vi "notemaker.vi"(11 "project-param in":T1) -> (3 "Reaper Note":string)   [LabVIEW 2019]
uses:
  Project Parameters.ctl
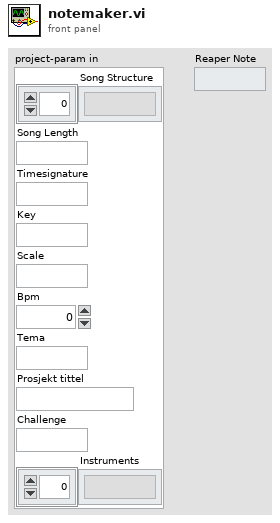
[diagram p1: front panel]
types:
  T1 = typedef "Project Parameters.ctl" = cluster{"Song Structure":string[], "Song Length":string, "Timesignature":string, "Key":string, "Scale":string, "Bpm":i32, "Tema":string, "Prosjekt tittel":string, "Challenge":string, "Instruments":string[]}
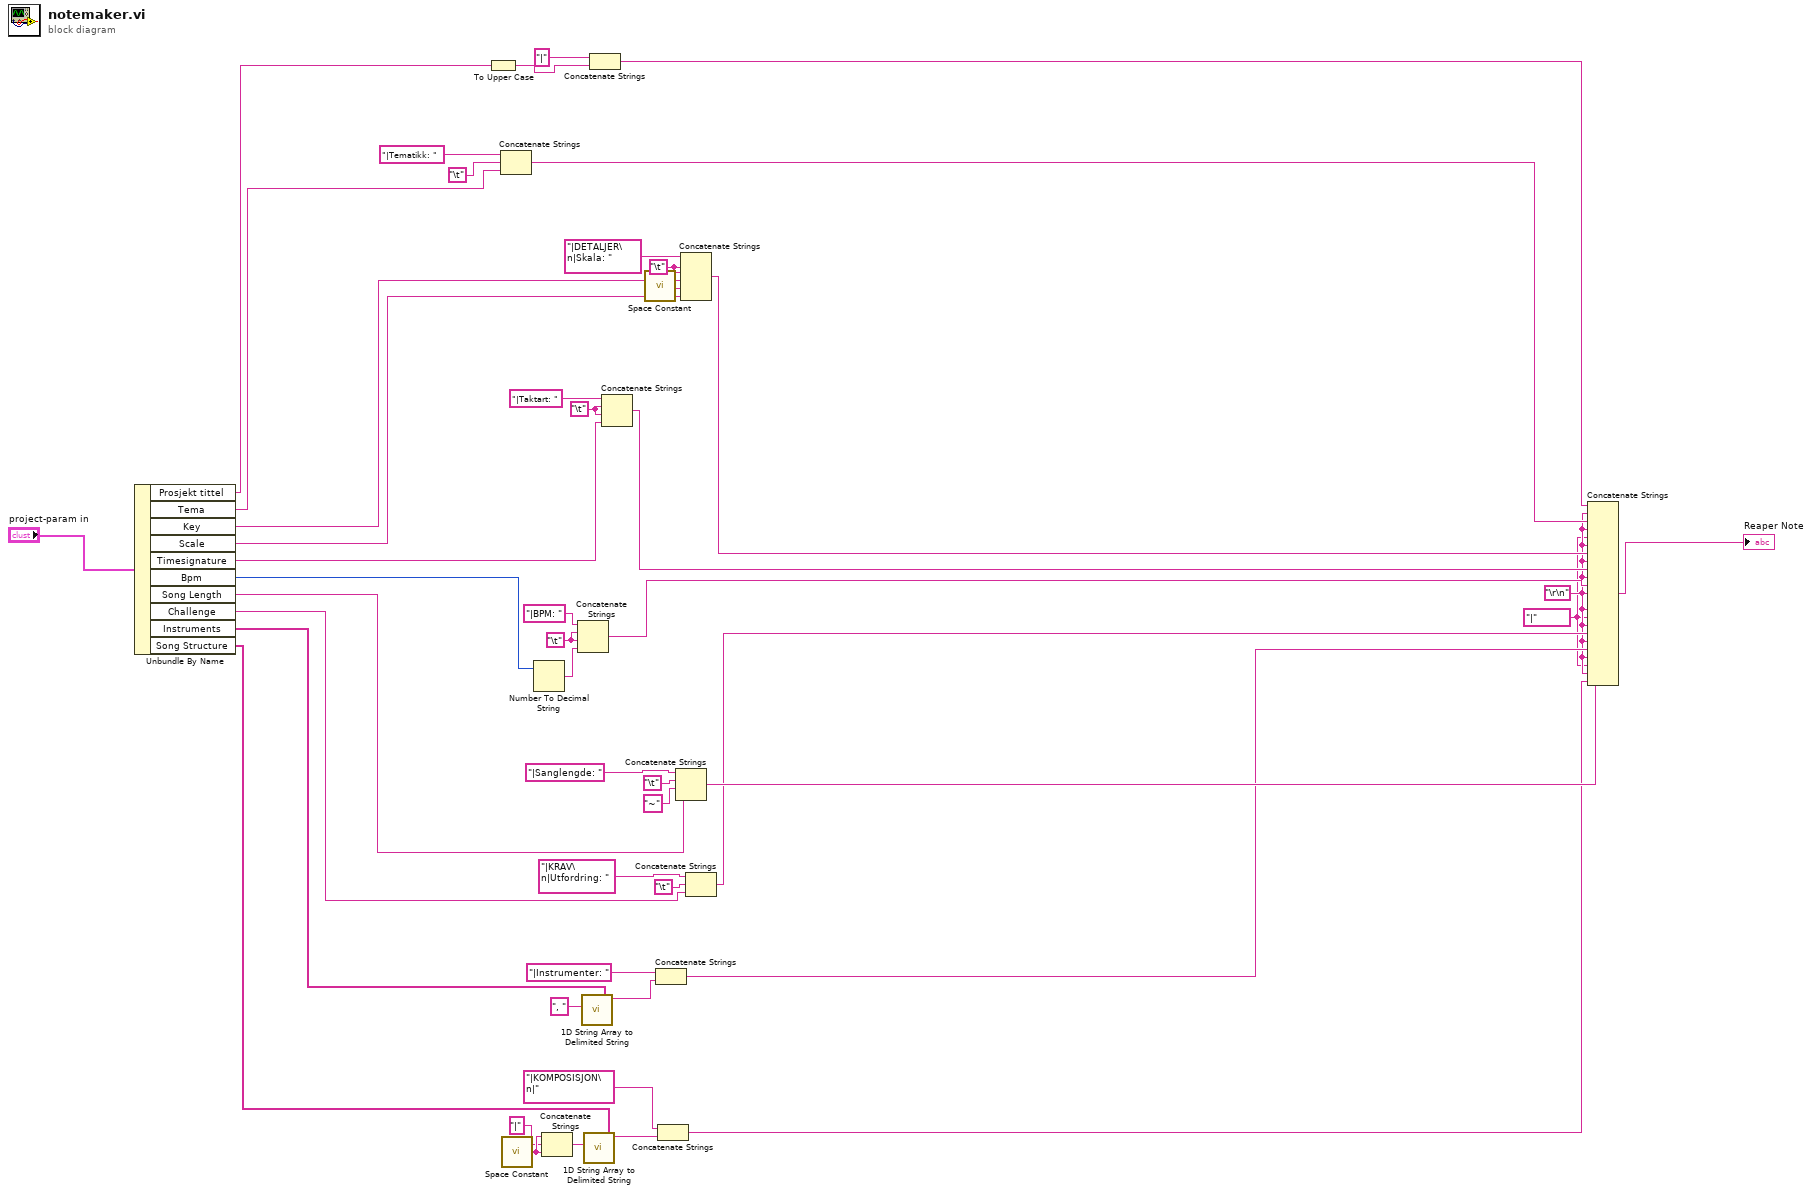
[diagram p0: block diagram]
diagram:
  w4 = "\t"
  w2 = "\t"
  w3 = "\t"
  w9 = "|" ("string")
  w10 = "\r\n"
  n1 = Unbundle By Name("project-param in") -> ("Prosjekt tittel"=w36:string, "Tema"=w11:string, "Key"=w33:string, "Scale"=w32:string, "Timesignature"=w31:string, "Bpm"=w46:i32, "Song Length"=w29:string, "Challenge"=w26:string, "Instruments"=w21:string[], "Song Structure"=w14:string[])
  n2 = To Upper Case(1:w36) -> (0:w37:string)
  n3 = Concatenate Strings("|Tematikk: " ("string"), "\t", w11) -> (w34:string)
  n4 = call <vilib>:"Space Constant.vi"() -> ("String"=w19:string)
  n5 = Number To Decimal String(number=w46) -> (decimal integer string=w47:string)  [unwired: 1 in]
  n6 = Concatenate Strings(w19, "|" ("string"), w19) -> (w20:string)
  n7 = Concatenate Strings("|BPM: " ("string"), w4, w4, w47) -> (w48:string)
  n8 = call <vilib>:"1D String Array to Delimited String.vi"("delimiter"=", " ("string"), "string array"=w21) -> ("delimited string"=w22:string)  [unwired: 9 in]
  n9 = call <vilib>:"1D String Array to Delimited String.vi"("delimiter"=w20, "string array"=w14) -> ("delimited string"=w15:string)  [unwired: 9 in]
  n10 = Concatenate Strings("|" ("string"), w37) -> (w13:string)
  n11 = Concatenate Strings("|Taktart: ", w3, w3, w31) -> (w43:string)
  n12 = call <vilib>:"Space Constant.vi"() -> ("String"=w40:string)
  n13 = Concatenate Strings("|Instrumenter: " ("string"), w22) -> (w23:string)
  n14 = Concatenate Strings("|KOMPOSISJON\n|" ("string"), w15) -> (w8:string)
  n15 = Concatenate Strings("|Sanglengde: " ("string"), "\t", "~" ("string"), w29) -> (w28:string)
  n16 = Concatenate Strings("|DETALJER\n|Skala: ", w2, w2, w33, w40, w32) -> (w41:string)
  n17 = Concatenate Strings("|KRAV\n|Utfordring: ", "\t", w26) -> (w25:string)
  n18 = Concatenate Strings(w13, w10, w34, w10, w9, w10, w41, w10, w43, w10, w48, w10, w28, w10, w9, w10, w25, w10, w23, w10, w9, w10, w8) -> (→"Reaper Note":string)
